vi "Compare Vector Length.vi"(10 "Vec 2":dbl[](array[numeric])=array[21000 elements], 11 "Vec 1":dbl[](array[numeric])=array[21000 elements]) -> (2 "Length(1) >= Length (2)":bool)   [LabVIEW 2021]
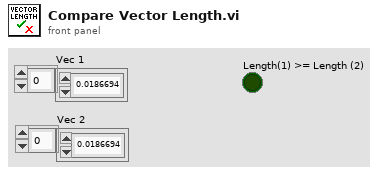
[diagram p1: front panel]
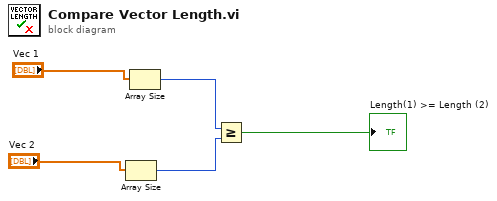
[diagram p0: block diagram]
diagram:
  n1 = Array Size(array="Vec 2") -> (size(s)=w2:i32)
  n2 = Array Size(array="Vec 1") -> (size(s)=w3:i32)
  n3 = Greater Or Equal?(x=w3, y=w2) -> (x >= y?=→"Length(1) >= Length (2)":bool)
